vi "Stats.vi"(0 "Analogue Data (volts)":dbl[][](array[numeric])) -> ()   [LabVIEW 2013]
uses:
  <vilib>/Analysis/NI_AALBase.lvlib
  <vilib>/gmath/NI_Gmath.lvlib
panel:
  out "Array":dbl[](array[numeric])
  out "array (last n elements first)":dbl[](array[numeric])
  out "Waveform Chart":dbl(graph)
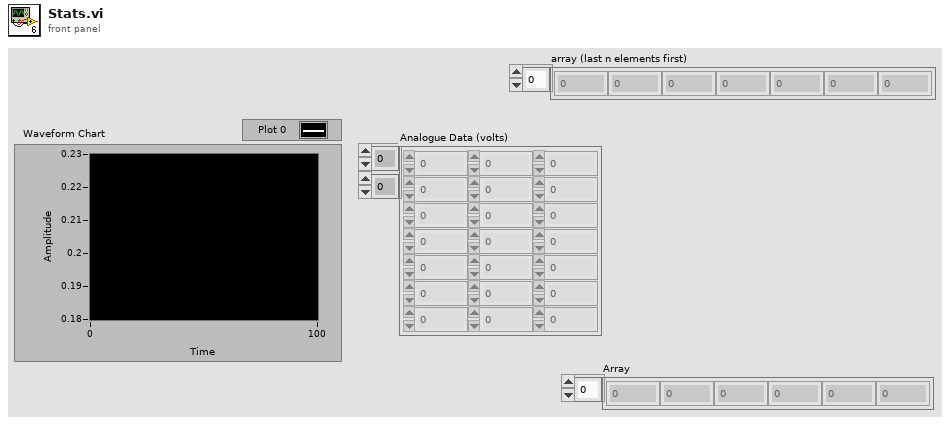
[diagram p1: front panel]
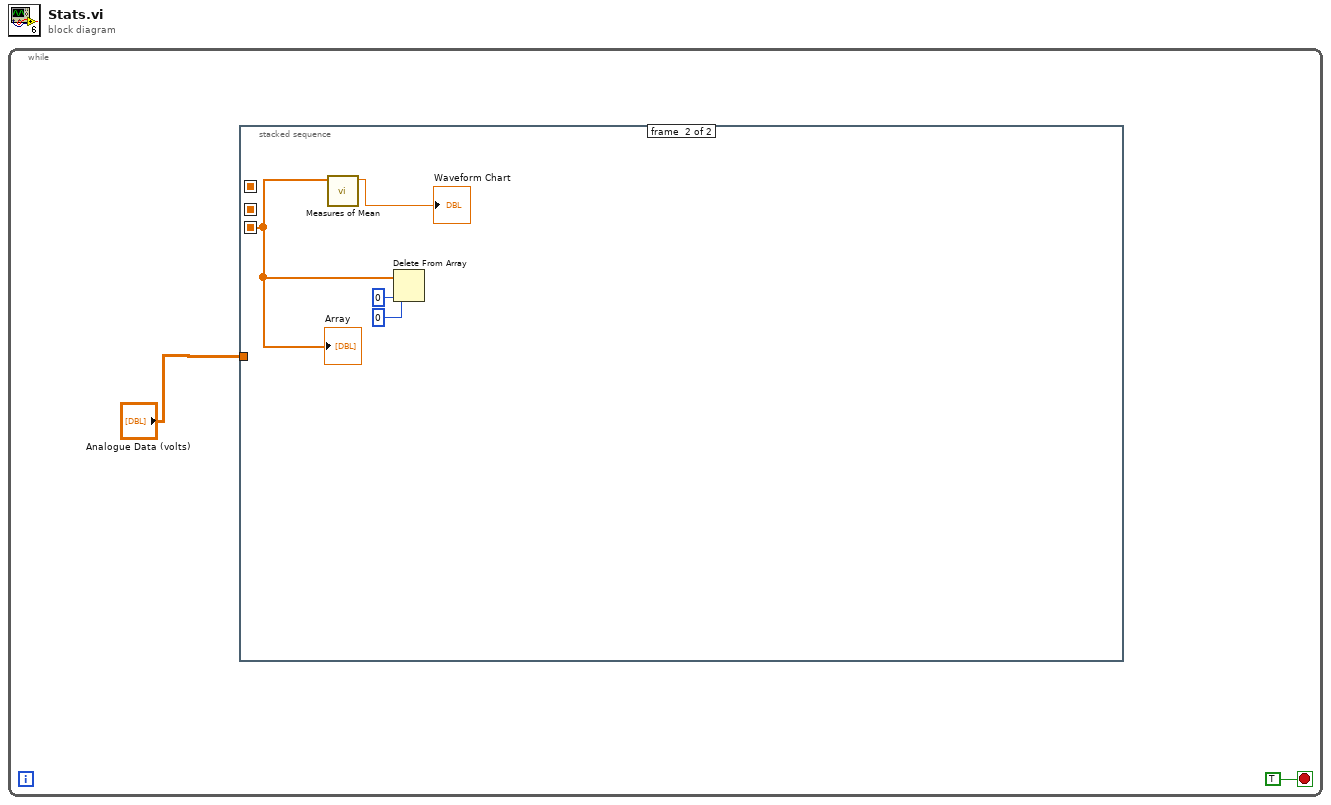
[diagram p0: block diagram]
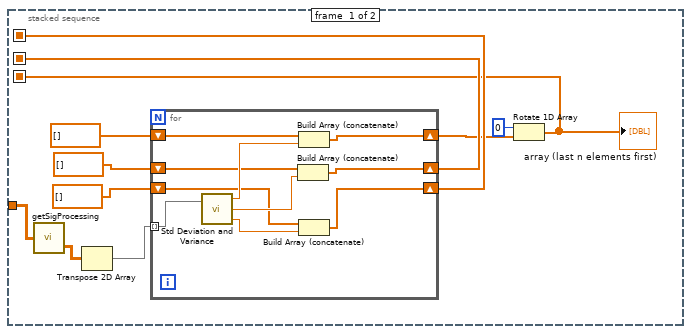
[diagram p2: hidden frame]
diagram:
  n1 = while {
    stop <- TRUE stop-if-true
    n2 = stacked-sequence {
      seq-local: [w3 _] -> [_ w26]
      seq-local: [w7 _] -> [_ _]
      seq-local: [w6 _] -> [_ _]
      tunnel: "Analogue Data (volts)" -> [w13 _]
      frame #0 {
        n3 = call "getSigProcessing.vi"("Analogue Data (volts)"=w13) -> ("Raw Signals"=w12:dbl[][])  [unwired: 1 out]
        n4 = Transpose 2D Array(2D array=w12) -> (transposed array=w11:dbl[][])
        n5 = for {
          tunnel: w11 -> [w22] mode=indexing
          shift-right: [w14] -> w4
          shift-left: dbl[] [] -> [w23]
          shift-right: [w17] -> w7
          shift-left: dbl[] [] -> [w18]
          shift-right: [w15] -> w6
          shift-left: dbl[] [] -> [w16]
          n6 = call <vilib>:"Std Deviation and Variance.vi"("X"=w22) -> ("mean"=w21:dbl, "standard deviation"=w20:dbl, "variance"=w19:dbl)  [unwired: 1 in]
          n7 = Build Array (concatenate)(w18, w20) -> (w17:dbl[])
          n8 = Build Array (concatenate)(w23, w21) -> (w14:dbl[])
          n9 = Build Array (concatenate)(w16, w19) -> (w15:dbl[])
        }
        n10 = Rotate 1D Array(1:w4, 2:0 ("n")) -> (0:w3:dbl[])
        "array (last n elements first)" <- w3
      }
      frame #1 {
        n11 = call <vilib>:"Measures of Mean.vi"("x array"=w26) -> ("mean value"=→"Waveform Chart":dbl)  [unwired: 9 in, 1 out]
        n12 = Delete From Array(array=w26, length=0, index=0) -> ()  [unwired: 2 out]
        "Array" <- w26
      }
    }
  }
